vi "Read Size of experimeents.vi"(8 "error in (no error)":errorcluster, 10 "Temp":bool, 11 "Experiment_merged in":refnum<class "Experiment_merged.lvclass">) -> (0 "error out":errorcluster, 2 "Size of experimeents":cluster{"X pixels":i32, "Y pixels":i32}[](array[cluster]), 3 "Experiment_merged out":refnum<class "Experiment_merged.lvclass">)   [LabVIEW 2020, in "Experiment_merged.lvclass"]
uses:
  Experiment_merged.lvclass
  Experiment_merged.lvclass/Experiment_merged.ctl
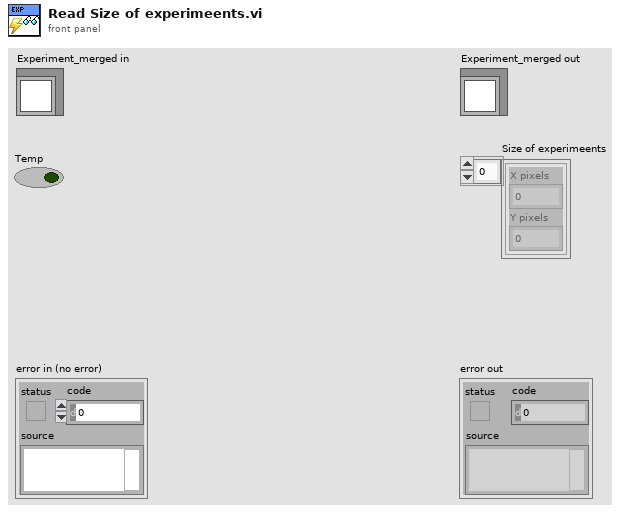
[diagram p1: front panel]
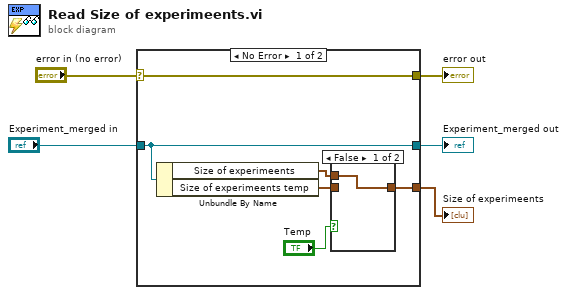
[diagram p0: block diagram]
diagram:
  n1 = case shown="No Error" "error in (no error)" {
    selector: "error in (no error)" -> [w11 w14]
    tunnel: [w11 w14] -> w4
    tunnel: [w10 w15] -> w2
    tunnel: "Experiment_merged in" -> [w10 w15]
    tunnel: [w8 _] -> w1
    frame No Error {
      n2 = Unbundle By Name(w10) -> ("Size of experimeents"=w6:cluster{"X pixels":i32, "Y pixels":i32}[], "Size of experimeents temp"=w7:cluster{"X pixels":i32, "Y pixels":i32}[])
      n3 = case shown="False" "Temp" {
        tunnel: [w12 w13] -> w8
        tunnel: w7 -> [_ w13]
        tunnel: w6 -> [w12 _]
        frame False {
        }
        frame True {
        }
      }
    }
    frame Error {
    }
  }
  "error out" <- w4
  "Experiment_merged out" <- w2
  "Size of experimeents" <- w1
